vi "Delta measure (SubVI).vi"(8 "错误输入（无错误）":errorcluster, 10 "config":refnum<queue>) -> (0 "错误输出":errorcluster, 3 "数组":string[](array[string]))   [LabVIEW 2019, in "SubVI.lvlib"]
uses:
  SubVI.lvlib
  config.ctl
  Instrument.ctl
  lib/QDInstrument.dll
  lib/Keithley 622x/Configure/Format/Typedefs/KE622x -- Optional Meas Elements.ctl
  KE7001.LLB/Keith 7001 Open/Close Chan.vi
  lib/Keithley 622x/Keithley 622x.lvlib
panel:
  # "(真是通道1，假是通道2)"
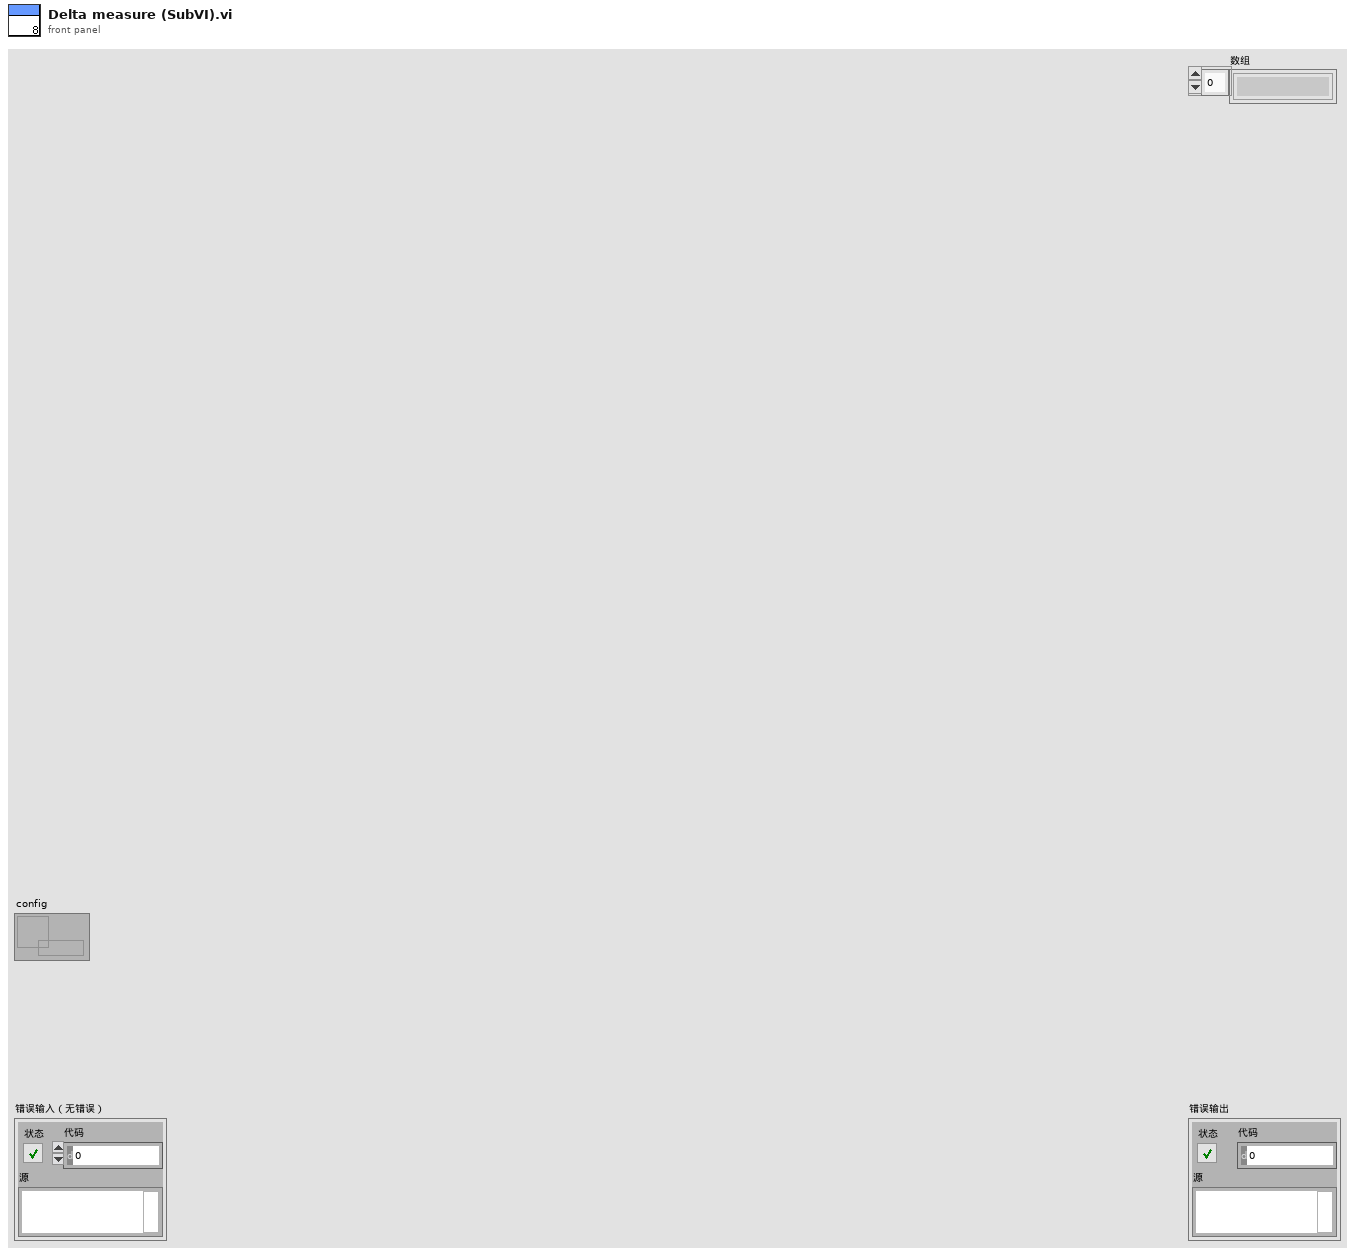
[diagram p1: front panel]
types:
  T1 = typedef "config.ctl" = cluster{"initialize":string, "6221":cluster{"6221 Resource":refnum<visa-resource-name>, "Delta status":bool}, "7001":cluster{"Ch":bool}, "SR830+6221":cluster{"source":u16, "阻抗":dbl, "量程入 4":i32, "量程入 3":i32, "量程入 2":i32, "量程入 1":i32, "电流":dbl, "SR830 2":bool, "SR830 3":bool, "SR830 4":bool, "SR830 1":bool, "VISA 1":refnum<visa-resource-name>, "VISA 2":refnum<visa-resource-name>, "VISA 3":refnum<visa-resource-name>, "VISA 4":refnum<visa-resource-name>, "量程":enum16{"量程每次测量会判定", "量程不变为设定值"}}, "2400":cluster{"2400":bool, "VISA":refnum<visa-resource-name>}, "ch":cluster{"ch str":string, "ch1":bool, "ch2":bool, "布尔":bool}, "error":bool, "数据文件路径":path, "log":cluster{"log路径":path, "log interval":dbl}, "Instrument":T2}
  T2 = typedef "Instrument.ctl" = cluster{"335 Resource":refnum<visa-resource-name>, "Input (0:A)":u16, "Instrument Type":i32, "quantum design":refnum<k24>, "Heater Output (1:1)":u16}
  T3 = cluster{"slot/memory":i16, "channel/row":i16, "column":i16, bool, bool}[]
  T4 = typedef "Keithley 622x.lvlib/KE622x -- Optional Meas Elements.ctl" = cluster{"Timstamp?":bool, "Reading Num?":bool, "Source Value?":bool, "Compliance?":bool, "Average Voltage?":bool}
  T5 = cluster{"error":bool, "code":i32, "source":string}
  T6 = typedef "Keithley 622x.lvlib/KE622x -- Meas Event Reg State.ctl" = cluster{"B0, ROF:  KE2182A Delta Reading Overflow Event?":bool, "B1, Int:  Interlock OK Event?":bool, "B2, Temp:  Over Temperature Event?":bool, "B3, Comp:  Compliance Event?":bool, "B5, RAV:  Delta Reading Available Event?":bool, "B6, TN:  User Defined Reading Number Stored In Buffer Event?":bool, "B7, BAV:  At Least 2 Readings Stored In Buffer Event?":bool, "B12, BQF:  Buffer Quarter Full Event?":bool, "B8, BHF:  Buffer Half Full Event?":bool, "B13, B3QF:  Buffer 3/4 Full Event?":bool, "B9, BFL:  Buffer Full Event?":bool}
  T7 = typedef "Keithley 622x.lvlib/KE622x -- Trace Buf.ctl" = cluster{"Additional Valid Arrays":T4, "Reading Num":u32[], "Timestamp (secs)":sgl[], "Source Val (A)":sgl[], "Reading":sgl[], "Average Voltage (V)":sgl[], "Compliance?":bool[]}
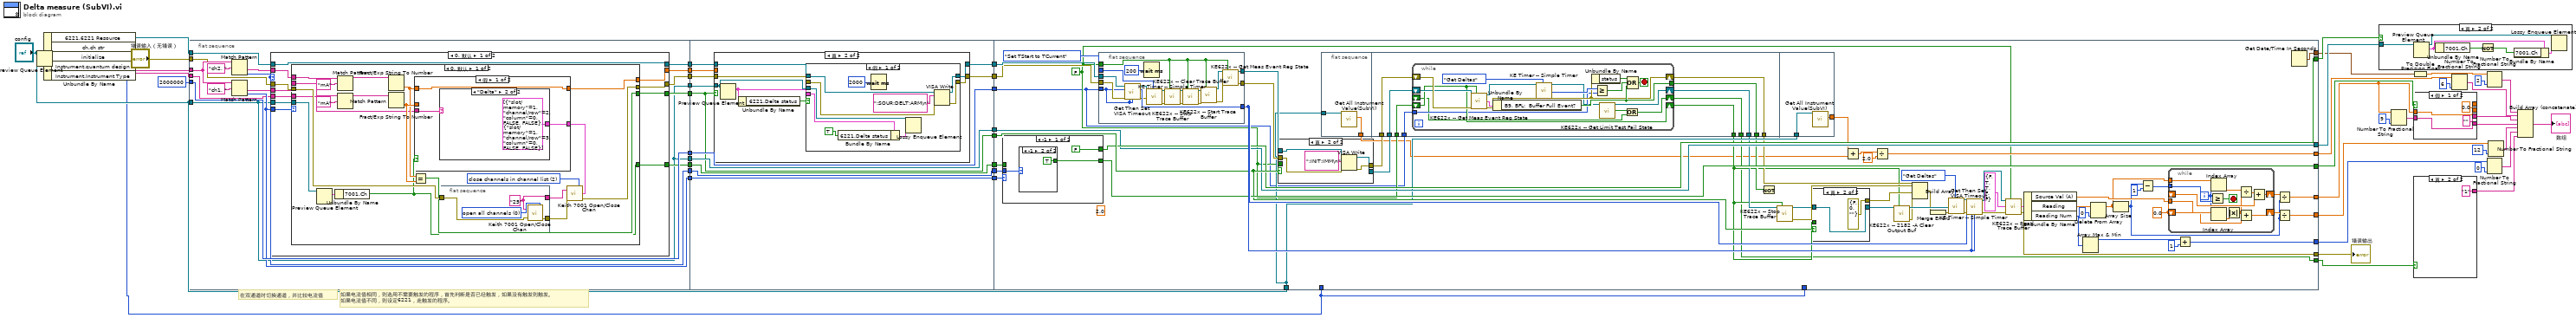
[diagram p0: block diagram]
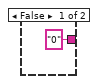
[diagram p2: hidden frame]
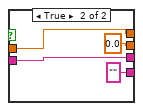
[diagram p4: hidden frame]
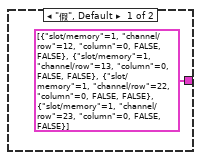
[diagram p5: hidden frame]
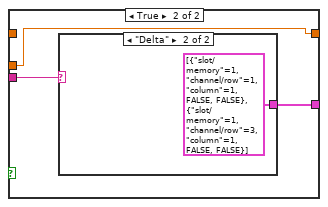
[diagram p6: hidden frame]
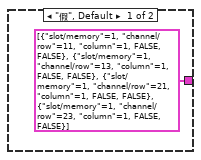
[diagram p7: hidden frame]
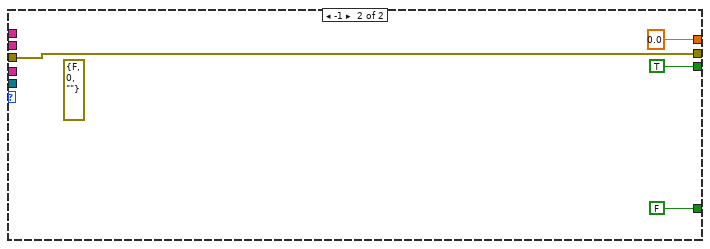
[diagram p8: hidden frame]
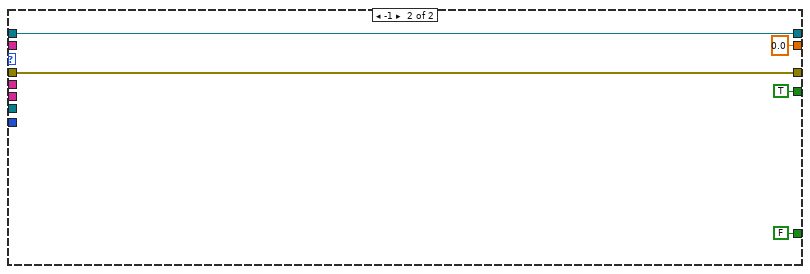
[diagram p9: hidden frame]
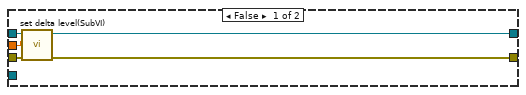
[diagram p10: hidden frame]
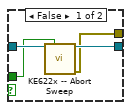
[diagram p12: hidden frame]
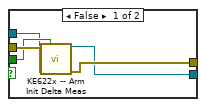
[diagram p13: hidden frame]
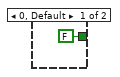
[diagram p14: hidden frame]
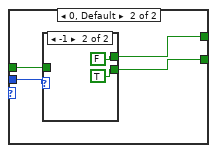
[diagram p15: hidden frame]
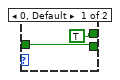
[diagram p16: hidden frame]
diagram:
  # "如果电流值相同，则选用不需要触发的程序，首先判断是否已经触发，如果没有触发则触发。\n如果电流值不同，则设定6221，走触发的程序。"
  # "在双通道时切换通道，并比较电流值"
  n1 = Preview Queue Element(queue="config") -> (element=w3:T1)  [unwired: 2 in, 3 out]
  n2 = Unbundle By Name(w3) -> ("6221.6221 Resource"=w25:refnum<visa-resource-name>, "ch.ch str"=w8:string, "initialize"=w7:string, "Instrument.Instrument Type"=w1:i32)  [unwired: 1 out]
  n3 = flat-sequence {
    tunnel: "config" -> [w52]
    tunnel: u32 2000000 ("Timeout (20000 ms)") -> [w68]
    tunnel: "错误输入（无错误）" -> [w58]
    tunnel: w25 -> [w65]
    tunnel: [w68] -> w51
    tunnel: [w52] -> w50
    tunnel: w8 -> [w64]
    tunnel: [w61] -> w49
    tunnel: [w60] -> w48
    tunnel: [w59] -> w47
    tunnel: [w57] -> w46
    tunnel: [w56] -> w45
    tunnel: [w55] -> w44
    tunnel: [w54] -> w43
    tunnel: w7 -> [w53]
    tunnel: [w52] -> w42
    tunnel: w51 -> [w134]
    tunnel: [w134] -> w41
    tunnel: w50 -> [w133]
    tunnel: [w133] -> w40
    tunnel: w49 -> [w132]
    tunnel: [w132] -> w39
    tunnel: w48 -> [w131]
    tunnel: [w131] -> w38
    tunnel: w47 -> [w130]
    tunnel: [w130] -> w37
    tunnel: w46 -> [w124]
    tunnel: w45 -> [w129]
    tunnel: w44 -> [w128]
    tunnel: w43 -> [w127]
    tunnel: [w126] -> w36
    tunnel: [w125] -> w35
    tunnel: [w124] -> w34
    tunnel: w42 -> [w123]
    tunnel: [w179] -> w9
    tunnel: [w200] -> w19
    tunnel: [w185] -> w18
    tunnel: [w194] -> w20
    tunnel: [w193] -> w33
    tunnel: w41 -> [w161]
    tunnel: w40 -> [w174]
    tunnel: [w184] -> w24
    tunnel: w39 -> [w183]
    tunnel: w38 -> [w182]
    tunnel: w37 -> [w181]
    tunnel: w36 -> [w192]
    tunnel: w35 -> [w203]
    tunnel: w34 -> [w180]
    tunnel: [w171] -> w26
    tunnel: [w175] -> w28
    tunnel: [w174] -> w29
    tunnel: [w162] -> w6
    tunnel: w1 -> [_]
    tunnel: "config" -> [w170]
    tunnel: w1 -> [_]
    frame #0 {
      n4 = Match Pattern(string=w64, regular expression="ch2, " ("正则表达式")) -> (after substring=w62:string, offset past match=w61:i32)  [unwired: 1 in, 2 out]
      n5 = Match Pattern(string=w64, regular expression="ch1, " ("正则表达式")) -> (after substring=w63:string, offset past match=w60:i32)  [unwired: 1 in, 2 out]
      n6 = case shown="0, 默认" w61 {
        tunnel: w65 -> [w71 w120]
        tunnel: w63 -> [w79 _]
        tunnel: w62 -> [w78 _]
        tunnel: w60 -> [w77 _]
        tunnel: [w76 FALSE ("create if not found? (T)")] -> w59
        tunnel: w58 -> [w75 w121]
        tunnel: [w74 TRUE] -> w57
        tunnel: [w73 w121] -> w56
        tunnel: [w72 0.0] -> w55
        tunnel: [w71 w120] -> w54
        tunnel: w53 -> [w70 _]
        tunnel: w52 -> [w69 _]
        frame 0, Default {
          n7 = case shown="0, 默认" w77 {
            tunnel: w79 -> [w93 _]
            tunnel: w78 -> [w95 _]
            tunnel: [w81 FALSE ("create if not found? (T)")] -> w76
            tunnel: w75 -> [w89 w115]
            tunnel: [w86 TRUE] -> w74
            tunnel: [w85 w115] -> w73
            tunnel: [w84 0.0] -> w72
            tunnel: w70 -> [w83 _]
            tunnel: w69 -> [w82 _]
            frame 0, Default {
              w98 = u16 2 items=["open all channels", "open channels in channel list", "close channels in channel list"] ("open/close (open all:0)")
              n8 = Preview Queue Element(queue=w82) -> (element=w80:T1)  [unwired: 2 in, 3 out]
              n9 = Unbundle By Name(w80) -> ("7001.Ch"=w81:bool)
              n10 = Match Pattern(string=w95, regular expression="mA" ("正则表达式")) -> (before substring=w90:string)  [unwired: 1 in, 3 out]
              n11 = Match Pattern(string=w93, regular expression="mA" ("正则表达式")) -> (before substring=w91:string)  [unwired: 1 in, 3 out]
              n12 = Fract/Exp String To Number(string=w90) -> (number=w87:dbl)  [unwired: 3 in, 1 out]
              n13 = Fract/Exp String To Number(string=w91) -> (number=w88:dbl)  [unwired: 3 in, 1 out]
              n14 = Equal?(x=w87, y=w88) -> (x = y?=w86:bool)
              n15 = case shown="假" w81 {
                tunnel: [w104 w109] -> w97
                tunnel: w88 -> [_ w111]
                tunnel: w87 -> [w106 _]
                tunnel: [w106 w111] -> w84
                tunnel: w83 -> [w105 w110]
                frame False {
                  n16 = case shown="\"Delta\"" w105 {
                    tunnel: [T3 [{"slot/memory"=1, "channel/row"=12, "column"=0, FALSE, FALSE}, {"slot/memory"=1, "channel/row"=13, "column"=0, FALSE, FALSE}, {"slot/memory"=1, "channel/row"=22, "column"=0, FALSE, FALSE}, {"slot/memory"=1, "channel/row"=23, "column"=0, FALSE, FALSE}] ("channel list") T3 [{"slot/memory"=1, "channel/row"=2, "column"=0, FALSE, FALSE}, {"slot/memory"=1, "channel/row"=3, "column"=0, FALSE, FALSE}] ("channel list")] -> w104
                    frame "假", Default {
                    }
                    frame "Delta" {
                    }
                  }
                }
                frame True {
                  n17 = case shown="\"Delta\"" w110 {
                    tunnel: [T3 [{"slot/memory"=1, "channel/row"=11, "column"=1, FALSE, FALSE}, {"slot/memory"=1, "channel/row"=13, "column"=1, FALSE, FALSE}, {"slot/memory"=1, "channel/row"=21, "column"=1, FALSE, FALSE}, {"slot/memory"=1, "channel/row"=23, "column"=1, FALSE, FALSE}] ("channel list") T3 [{"slot/memory"=1, "channel/row"=1, "column"=1, FALSE, FALSE}, {"slot/memory"=1, "channel/row"=3, "column"=1, FALSE, FALSE}] ("channel list")] -> w109
                    frame "假", Default {
                    }
                    frame "Delta" {
                    }
                  }
                }
              }
              n18 = flat-sequence {
                tunnel: [w102] -> w99
                tunnel: [w101] -> w96
                tunnel: w89 -> [w100]
                frame #0 {
                  w103 = u16 0 items=["open all channels", "open channels in channel list", "close channels in channel list"] ("open/close (open all:0)")
                  w102 = "25" ("GPIB address")
                  n19 = call "Keith 7001 Open/Close Chan.vi"("GPIB address"=w102, "error in"=w100, "open/close (open all:0)"=w103) -> ("error out"=w101:T5)  [unwired: 1 in]
                }
              }
              n20 = call "Keith 7001 Open/Close Chan.vi"("GPIB address"=w99, "error in"=w96, "open/close (open all:0)"=w98, "channel list"=w97) -> ("error out"=w85:T5)
            }
            frame -1 {
              (unwired) errorcluster {"status"=FALSE, "code"=0, "source"=""} ("错误输出")
            }
          }
        }
        frame -1 {
        }
      }
    }
    frame #1 {
      n21 = case shown="真" w124 {
        tunnel: w129 -> [w139 w145]
        tunnel: w128 -> [w138 _]
        tunnel: w127 -> [w137 w146]
        tunnel: [w136 w144] -> w125
        tunnel: [w135 w143] -> w126
        tunnel: w123 -> [_ w140]
        frame False {
          n22 = call "set delta level(SubVI).vi"("错误输入（无错误）"=w139, "电流（A）"=w138, "VISA引用句柄输入"=w137) -> ("错误输出"=w135:errorcluster, "VISA引用句柄输出"=w136:refnum<visa-resource-name>)  [unwired: 7 in]
        }
        frame True {
          n23 = Preview Queue Element(queue=w140) -> (element=w141:T1)  [unwired: 2 in, 3 out]
          n24 = Unbundle By Name(w141) -> ("6221.Delta status"=w142:bool)
          n25 = case shown="假" w142 {
            tunnel: w146 -> [w152 w157]
            tunnel: [w153 w157] -> w144
            tunnel: w145 -> [w155 w158]
            tunnel: [w154 w158] -> w143
            tunnel: w141 -> [w149 _]
            tunnel: w140 -> [w148 _]
            frame False {
              n26 = Bundle By Name(cluster=w149, "6221.Delta status"=TRUE) -> (w147:T1)
              n27 = Wait (ms)(milliseconds to wait=u32 2000) -> ()  [unwired: 1 out]
              n28 = Lossy Enqueue Element(queue=w148, element=w147) -> ()  [unwired: 1 in, 4 out]
              n29 = VISA Write(VISA resource name=w152, write buffer=":SOUR:DELT:ARM\n" ("format string"), error in (no error)=w155) -> (VISA resource name out=w153:refnum<visa-resource-name>, error out=w154:errorcluster)  [unwired: 1 out]
            }
            frame True {
            }
          }
        }
      }
    }
    frame #2 {
      w167 = FALSE ("Check For SCPI Errors? (T) 2")
      (unwired) 2.0 ("y")
      w198 = sgl 0.0 ("Numeric")
      n30 = case shown="-1" w182 {
        tunnel: [w289 w295] -> w184
        tunnel: w183 -> [w288 w294]
        tunnel: w181 -> [_ w293]
        tunnel: [FALSE w292] -> w175
        frame -1 {
          n31 = case shown="-1" w288 {
            tunnel: [FALSE TRUE] -> w289
            frame 0, Default {
            }
            frame -1 {
            }
          }
        }
        frame 0, Default {
          n32 = case shown="-1" w294 {
            tunnel: [w297 TRUE] -> w295
            tunnel: w293 -> [w297 _]
            tunnel: [TRUE FALSE] -> w292
            frame 0, Default {
            }
            frame -1 {
            }
          }
        }
      }
      n33 = flat-sequence {
        tunnel: enum16{"Set TStart to TCurrent", "Get Deltas"}."Set TStart to TCurrent" ("Action") -> [w266]
        tunnel: [w263] -> w212
        tunnel: [w262] -> w211
        tunnel: [w259] -> w204
        tunnel: w203 -> [w256]
        tunnel: w167 -> [w255]
        tunnel: w192 -> [w254]
        tunnel: w161 -> [w253]
        frame #0 {
          n34 = call "Get Then Set VISA Timeout.vi"("VISA Resource Name In"=w256, "New Timeout (msecs)"=w253, "error in (no error)"=w254, "Max Timeout (300 secs)"=w253, "Min Timeout (3 secs)"=w253) -> ("VISA Resource Name Out (dupl)"=w258:refnum<visa-resource-name>, "Old Timeout (msecs)"=w259:u32, "error out"=w257:errorcluster)  [unwired: 7 in, 1 out]
          n35 = Wait (ms)(milliseconds to wait=u32 200) -> ()  [unwired: 1 out]
          n36 = call "KE Timer -- Simple Timer.vi"("Resource In"=w258, "error in (no error)"=w257, "Action"=w266) -> ("Resource Out (dupl)"=w265:refnum<visa-resource-name>, "error out (dupl)"=w264:errorcluster)  [unwired: 7 in, 8 out]
          n37 = call "KE622x -- Stop Trace Buffer.vi"("Resource In"=w265, "Check For SCPI Errors? (T)"=w255, "error in (no error)"=w264) -> ("Resource Out (dupl)"=w270:refnum<visa-resource-name>, "error out"=w269:errorcluster)  [unwired: 11 in]
          n38 = call "KE622x -- Clear Trace Buffer.vi"("Resource In"=w270, "Check For SCPI Errors? (T)"=w255, "error in (no error)"=w269) -> ("Resource Out (dupl)"=w261:refnum<visa-resource-name>, "error out"=w260:errorcluster)  [unwired: 11 in]
          n39 = call "KE622x -- Start Trace Buffer.vi"("Resource In"=w261, "Check For SCPI Errors? (T)"=w255, "error in (no error)"=w260) -> ("Resource Out (dupl)"=w267:refnum<visa-resource-name>, "error out"=w268:errorcluster)  [unwired: 11 in]
          n40 = call "KE622x -- Get Meas Event Reg State.vi"("VISA Resource In"=w267, "Error Query (T)?"=w255, "error in (no error)"=w268) -> ("VISA Resource Out (dupl)"=w263:refnum<visa-resource-name>, "error out"=w262:errorcluster)  [unwired: 10 in, 1 out]
        }
      }
      n41 = case shown="真" w180 {
        tunnel: [w281 w283] -> w169
        tunnel: [w280 w282] -> w168
        tunnel: w212 -> [w277 w285]
        tunnel: w211 -> [w279 w284]
        tunnel: w167 -> [w278 _]
        frame False {
          n42 = call "KE622x -- Arm Init Delta Meas.vi"("Resource In"=w277, "Check For SCPI Errors? (T)"=w278, "error in (no error)"=w279) -> ("Resource Out (dupl)"=w280:refnum<visa-resource-name>, "error out"=w281:errorcluster)  [unwired: 11 in]
        }
        frame True {
          n43 = VISA Write(VISA resource name=w285, write buffer=":INIT:IMM\n", error in (no error)=w284) -> (VISA resource name out=w282:refnum<visa-resource-name>, error out=w283:errorcluster)  [unwired: 1 out]
        }
      }
      n44 = flat-sequence {
        tunnel: w170 -> [w221]
        tunnel: [w220] -> w159
        tunnel: w169 -> [w230]
        tunnel: w168 -> [w229]
        tunnel: w167 -> [w228]
        tunnel: [w227] -> w166
        tunnel: [w226] -> w165
        tunnel: [w225] -> w164
        tunnel: [w224] -> w163
        tunnel: [w223] -> w162
        tunnel: w161 -> [w222]
        tunnel: w170 -> [w251]
        tunnel: [w250] -> w160
        frame #0 {
          n45 = call "Get All Instrument Value(SubVI).vi"("队列输入"=w221) -> ("数组"=w220:dbl[])  [unwired: 10 in]
        }
        frame #1 {
          n46 = while {
            shift-right: [w238] -> w227
            shift-left: w230 -> [w249]
            shift-right: [w234] -> w226
            shift-left: w229 -> [w248]
            tunnel: [w241] -> w225
            shift-right: [w239] -> w224
            shift-left: w228 -> [w239]
            tunnel: w222 -> [w236]
            shift-right: [w232] -> w223
            shift-left: _ -> [w231]
            stop <- w242 stop-if-true
            n47 = call "KE622x -- Get Meas Event Reg State.vi"("VISA Resource In"=w248, "Error Query (T)?"=w239, "error in (no error)"=w249) -> ("VISA Resource Out (dupl)"=w245:refnum<visa-resource-name>, "KE622x Meas Event Reg"=w247:T6, "error out"=w246:errorcluster)  [unwired: 10 in]
            n48 = Unbundle By Name(w247) -> ("B9, BFL:  Buffer Full Event?"=w241:bool)
            n49 = call "KE Timer -- Simple Timer.vi"("Resource In"=w245, "error in (no error)"=w246, "Action"=enum16{"Set TStart to TCurrent", "Get Deltas"}."Get Deltas") -> ("Resource Out (dupl)"=w235:refnum<visa-resource-name>, "TCurrent - TStart (ms)"=w243:u32, "error out (dupl)"=w238:errorcluster)  [unwired: 7 in, 7 out]
            n50 = Unbundle By Name(w238) -> ("status"=w237:bool)
            n51 = Greater Or Equal?(x=w243, y=w236) -> (x >= y?=w240:bool)
            n52 = call "KE622x -- Get Limit Test Fail State.vi"("Resource In"=w235) -> ("Resource Out (dupl)"=w234:refnum<visa-resource-name>, "Limit Test Failed (Compliance)?"=w233:bool)  [unwired: 12 in, 1 out]
            n53 = Or(x=w233, y=w231) -> (x .or. y?=w232:bool)
            n54 = Compound Arithmetic op=OR(w237, w240, w241) -> (w242:bool)
          }
        }
        frame #2 {
          n55 = call "Get All Instrument Value(SubVI).vi"("队列输入"=w251) -> ("数组"=w250:dbl[])  [unwired: 10 in]
        }
      }
      n56 = Not(x=w164) -> ()  [unwired: 1 out]
      n57 = call "KE622x -- Stop Trace Buffer.vi"("Resource In"=w165, "Check For SCPI Errors? (T)"=w163) -> ("Resource Out (dupl)"=w191:refnum<visa-resource-name>, "error out"=w209:errorcluster)  [unwired: 12 in]
      n58 = case shown="真" w180 {
        tunnel: w163 -> [w273 _]
        tunnel: [w272 w276] -> w190
        tunnel: [w271 errorcluster {"status"=FALSE, "code"=0, "source"=""} ("error out")] -> w189
        tunnel: w191 -> [w274 w276]
        frame False {
          n59 = call "KE622x -- Abort Sweep.vi"("Resource In"=w274, "Check For SCPI Errors? (T)"=w273) -> ("Resource Out (dupl)"=w272:refnum<visa-resource-name>, "error out"=w271:errorcluster)  [unwired: 12 in]
        }
        frame True {
        }
      }
      n60 = Add(x=w160, y=w159) -> (x+y=w173:dbl[])
      n61 = Divide(x=w173, y=2.0) -> (x/y=w171:dbl[])
      n62 = call "KE622x -- 2182 -A Clear Output Buf.vi"("622x Resource In"=w190, "Check For SCPI Errors? (T)"=w163) -> ("622x Resource Out (dupl)"=w214:refnum<visa-resource-name>, "error out"=w208:errorcluster)  [unwired: 11 in, 1 out]
      n63 = Build Array(w166, w209, w189, w208) -> (w210:errorcluster[])
      n64 = Merge Errors(w210) -> (w207:errorcluster)
      n65 = call "KE Timer -- Simple Timer.vi"("Resource In"=w214, "error in (no error)"=w207, "Action"=enum16{"Set TStart to TCurrent", "Get Deltas"}."Get Deltas") -> ("Resource Out (dupl)"=w205:refnum<visa-resource-name>, "error out (dupl)"=w206:errorcluster)  [unwired: 7 in, 8 out]
      n66 = call "Get Then Set VISA Timeout.vi"("VISA Resource Name In"=w205, "New Timeout (msecs)"=w204, "error in (no error)"=w206, "Max Timeout (300 secs)"=w204, "Min Timeout (3 secs)"=w204) -> ("VISA Resource Name Out (dupl)"=w202:refnum<visa-resource-name>, "error out"=w201:errorcluster)  [unwired: 7 in, 2 out]
      n67 = call "KE622x -- Read Trace Buffer.vi"("Resource In"=w202, "Check For SCPI Errors? (T)"=w167, "Meas Elements To Return"=T4 {"Timstamp?"=FALSE, "Reading Num?"=TRUE, "Source Value?"=TRUE, "Compliance?"=FALSE, "Average Voltage?"=FALSE}, "error in (no error)"=w201) -> ("Trace Buf"=w219:T7, "error out"=w193:errorcluster)  [unwired: 9 in, 1 out]
      n68 = Unbundle By Name(w219) -> ("Source Val (A)"=w196:sgl[], "Reading"=w177:sgl[], "Reading Num"=w199:u32[])
      n69 = Array Max & Min(array=w199) -> (max value=w187:u32)  [unwired: 3 out]
      n70 = Delete From Array(array=w177, index=0 ("索引")) -> (array with subset deleted=w176:sgl[])  [unwired: 1 in, 1 out]
      n71 = Array Size(array=w176) -> (size(s)=w195:i32)
      n72 = Subtract(x=w195, y=1) -> (x-y=w216:i32)
      n73 = while {
        tunnel: w176 -> [w312]
        shift-right: [w310] -> w218
        shift-left: w198 -> [w311]
        tunnel: w216 -> [w309]
        tunnel: w196 -> [w307]
        shift-right: [w304] -> w197
        shift-left: w198 -> [w305]
        i -> [w306]
        stop <- w308 stop-if-true
        n74 = Greater Or Equal?(x=w306, y=w309) -> (x >= y?=w308:bool)
        n75 = Index Array(array=w312, index=w306) -> (element=w303:sgl)
        n76 = Index Array(array=w307, index=w306) -> (element=w302:sgl)
        n77 = Absolute Value(x=w302) -> (abs(x)=w300:sgl)
        n78 = Divide(x=w303, y=w300) -> (x/y=w301:sgl)
        n79 = Add(x=w300, y=w305) -> (x+y=w304:sgl)
        n80 = Add(x=w301, y=w311) -> (x+y=w310:sgl)
      }
      n81 = Add(x=w187, y=u32 1) -> (x+y=w185:u32)
      n82 = Divide(x=w218, y=w195) -> (x/y=w200:sgl)
      n83 = Divide(x=w197, y=w195) -> (x/y=w194:sgl)
      n84 = Get Date/Time In Seconds() -> (seconds since 1Jan1904=w179:timestamp)
    }
  }
  n85 = case shown="真" w28 {
    tunnel: w29 -> [_ w318]
    frame False {
    }
    frame True {
      n86 = Preview Queue Element(queue=w318) -> (queue out=w313:refnum<queue>, element=w316:T1)  [unwired: 2 in, 2 out]
      n87 = Unbundle By Name(w316) -> ("7001.Ch"=w317:bool)
      n88 = Not(x=w317) -> (.not. x?=w315:bool)
      n89 = Bundle By Name(cluster=w316, "7001.Ch"=w315) -> (w314:T1)
      n90 = Lossy Enqueue Element(queue=w313, element=w314) -> ()  [unwired: 1 in, 4 out]
    }
  }
  n91 = Number To Fractional String(number=w19, precision (6)=i16 9 ("精度(6)")) -> (F-format string=w14:string)  [unwired: 2 in]
  n92 = To Double Precision Float(number=w9) -> (double precision float=w10:dbl)
  n93 = case shown="假" w24 {
    tunnel: [sgl 0.0 w326] -> _
    tunnel: w19 -> [w322 w326]
    tunnel: [w322 0.0 ("元素")] -> _
    tunnel: w14 -> [w319 w324]
    tunnel: ["" w324] -> w15
    tunnel: [w319 ""] -> w16
    frame False {
    }
    frame True {
    }
  }
  n94 = case shown="真" w6 {
    tunnel: ["0" "1"] -> w4
    frame False {
    }
    frame True {
    }
  }
  n95 = Number To Fractional String(number=w26, precision (6)=i16 6 ("精度(6)")) -> (F-format string=w5:string[])  [unwired: 2 in]
  n96 = Number To Fractional String(number=w10, precision (6)=i16 2 ("精度(6)")) -> (F-format string=w12:string)  [unwired: 2 in]
  n97 = Number To Fractional String(number=w18, precision (6)=i16 0 ("精度(6)")) -> (F-format string=w22:string)  [unwired: 2 in]
  n98 = Number To Fractional String(number=w20, precision (6)=i16 12) -> (F-format string=w23:string)  [unwired: 2 in]
  n99 = Build Array (concatenate)(w12, w5, w15, w16, w23, w22, w4) -> (→"数组":string[])
  "错误输出" <- w33
